vi "PosNegOddEven.vi"() -> ()   [LabVIEW 2021]
panel:
  out "String 5":string
  in  "String 4":string
  in  "String 3":string
  in  "String 2":string
  in  "String":string
  in  "A":dbl
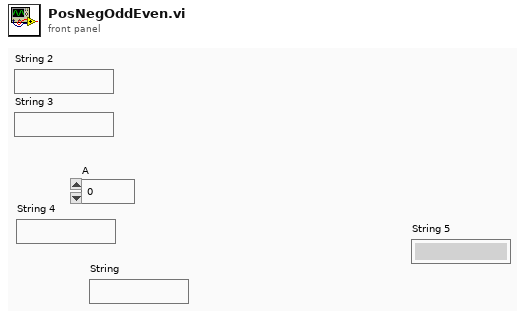
[diagram p1: front panel]
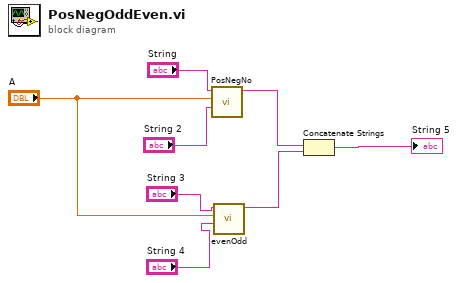
[diagram p0: block diagram]
diagram:
  n1 = call "PosNegNo.vi"("String 2"="String 2", "A"="A", "String"="String") -> ("String 3"=w3:string)  [unwired: 8 in]
  n2 = call "evenOdd.vi"("String 2"="String 4", "A"="A", "String"="String 3") -> ("String 3"=w2:string)  [unwired: 8 in]
  n3 = Concatenate Strings(w3, w2) -> (→"String 5":string)
